vi "Datasheet Find Data.vi"(5 "SN":string, 6 "Test Type":string, 7 "MN":string, 8 "error in (no error)":errorcluster, 10 "Run Information":T2, 11 "Column Data":T1) -> (0 "error out":errorcluster, 3 "Column Item":string)   [LabVIEW 2011]
uses:
  TDMS/TDMS Run.ctl
  TDMS/TDMS Channel (Sxx).ctl
  database/Fields/Field Record.ctl
  database/Fields/Field DataTypes.ctl
  database/Fields/Field NextItem.ctl
  Column Data.ctl
  www/tests/S Parameter/TypeDefs/SP Format.ctl
  Datasheet Table Sxx Type.ctl
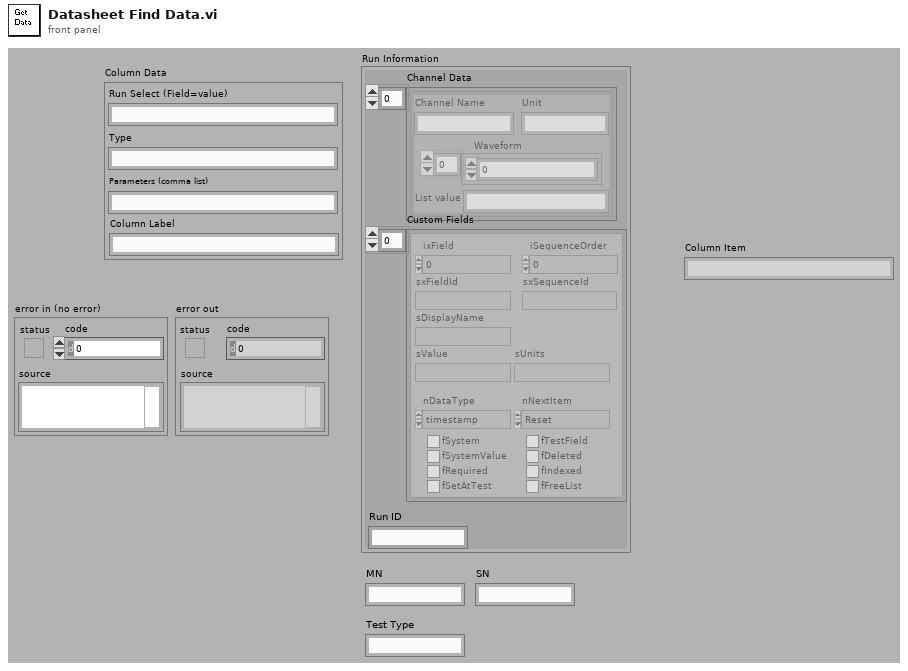
[diagram p1: front panel]
types:
  T1 = typedef "Column Data.ctl" = cluster{"Run Select (Field=value)":string, "Type":string, "Parameters (comma list)":string, "Column Label":string}
  T2 = typedef "TDMS Run.ctl" = cluster{"Channel Data":T3[], "Custom Fields":T4[], "Run ID":string}
  T3 = typedef "TDMS Channel (Sxx).ctl" = cluster{"Channel Name":string, "Waveform":dbl[], "Unit":string, "List value":string}
  T4 = typedef "Field Record.ctl" = cluster{"ixField":i32, "iSequenceOrder":i32, "sxFieldId":string, "sxSequenceId":string, "sDisplayName":string, "sValue":string, "sUnits":string, "nDataType":T5, "nNextItem":T6, "fSystem":bool, "fSystemValue":bool, "fRequired":bool, "fSetAtTest":bool, "fTestField":bool, "fDeleted":bool, "fIndexed":bool, "fFreeList":bool}
  T5 = typedef "Field DataTypes.ctl" = enum32{"text", "numeric", "list", "timestamp", "boolean"}
  T6 = typedef "Field NextItem.ctl" = enum32{"Reset", "Retain", "Auto-Increment"}
  T7 = typedef "datasheet table Sxx type.ctl" = enum16{"Value", "Maximum", "Minimum", "Max Freq", "maxlimit", "minlimit", "Min Freq", "maxfreqlimit", "minfreqlimit"}
  T8 = typedef "SP Format.ctl" = enum16{"Log Mag", "Lin Mag", "SWR", "Phase", "Expanded Phase", "Delay", "Insertion Loss", "Isolation", "Return Loss"}
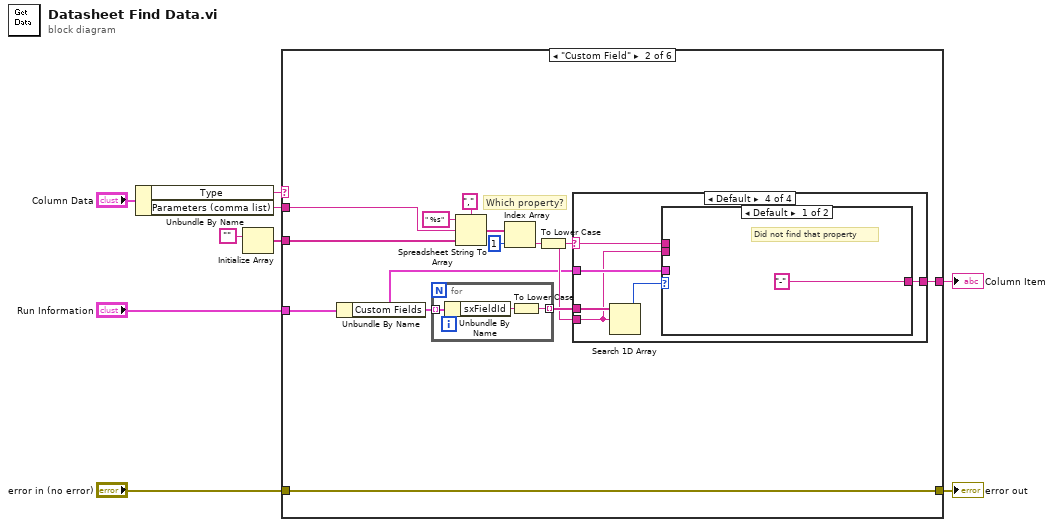
[diagram p0: block diagram]
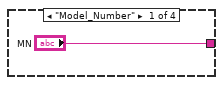
[diagram p3: hidden frame]
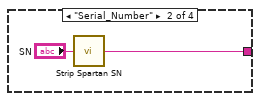
[diagram p4: hidden frame]
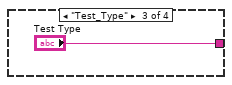
[diagram p5: hidden frame]
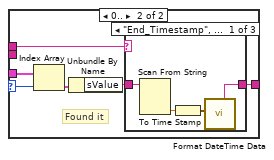
[diagram p6: hidden frame]
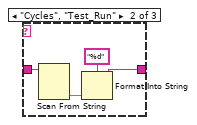
[diagram p7: hidden frame]
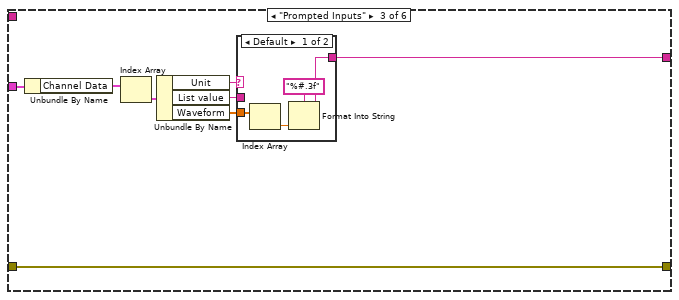
[diagram p9: hidden frame]
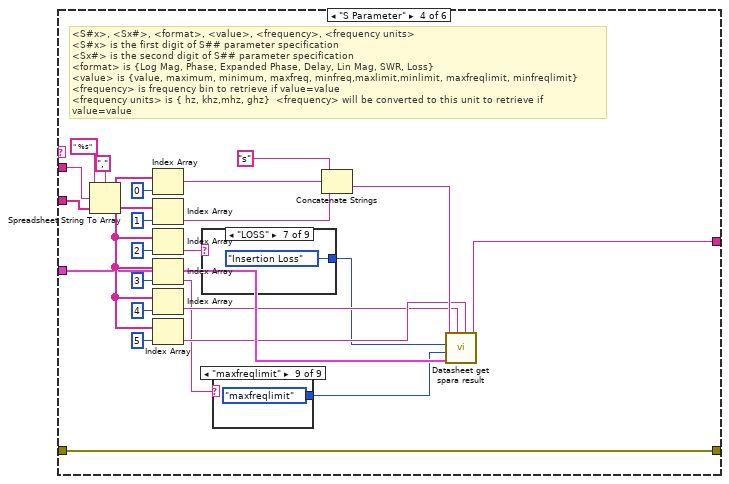
[diagram p11: hidden frame]
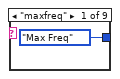
[diagram p12: hidden frame]
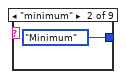
[diagram p13: hidden frame]
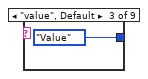
[diagram p14: hidden frame]
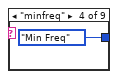
[diagram p15: hidden frame]
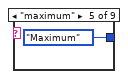
[diagram p16: hidden frame]
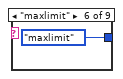
[diagram p17: hidden frame]
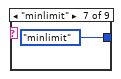
[diagram p18: hidden frame]
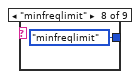
[diagram p19: hidden frame]
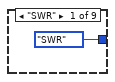
[diagram p20: hidden frame]
diagram:
  n1 = Unbundle By Name("Column Data") -> ("Type"=w8:string, "Parameters (comma list)"=w7:string)
  n2 = Initialize Array("") -> (w6:string[])  [unwired: 1 out]
  n3 = case shown="\"Custom Field\"" w8 {
    tunnel: w7 -> [w11 w21 _ w89 w121 w133]
    tunnel: w6 -> [_ w20 _ w88 w120 w132]
    tunnel: "Run Information" -> [_ w19 w60 w84 w109 w131]
    tunnel: [w11 w17 w55 w83 w116 w128] -> w3
    tunnel: "error in (no error)" -> [w10 w15 w61 w86 w118 w125]
    tunnel: [w10 w15 w61 w86 w118 w125] -> w1
    frame Default {
    }
    frame "Custom Field" {
      # "Which property?"
      n4 = Unbundle By Name(w19) -> ("Custom Fields"=w12:T4[])
      n5 = for {
        tunnel: w12 -> [w53] mode=indexing
        tunnel: [w51] -> w18 mode=indexing
        n6 = Unbundle By Name(w53) -> ("sxFieldId"=w52:string)
        n7 = To Lower Case(string=w52) -> (all lower case string=w51:string)
      }
      n8 = Spreadsheet String To Array(delimiter (Tab)=",", format string=" %s" ("delimiter (Tab)"), spreadsheet string=w21, array type (2D Dbl)=w20) -> (array=w22:string[])
      n9 = Index Array(array=w22, index=1) -> (element=w14:string)
      n10 = To Lower Case(string=w14) -> (all lower case string=w13:string)
      n11 = case shown="Default" w13 {
        selector: w13 -> [_ _ _ w29]
        tunnel: w18 -> [_ _ _ w34]
        tunnel: ["MN" w26 "Test Type" w32] -> w17
        tunnel: w12 -> [_ _ _ w31]
        tunnel: w13 -> [_ _ _ w30]
        frame "Model_Number" {
        }
        frame "Serial_Number" {
          n12 = call "Strip Spartan SN.vi"("SN 2"="SN") -> ("SN"=w26:string)
        }
        frame "Test_Type" {
        }
        frame Default {
          n13 = Search 1D Array(1D array=w34, element=w30) -> (index of element=w33:i32)  [unwired: 1 out]
          n14 = case shown="Default" w33 {
            selector: w33 -> [_ w40]
            tunnel: ["-" w36] -> w32
            tunnel: w31 -> [_ w41]
            tunnel: w30 -> [_ _]
            tunnel: w29 -> [_ w38]
            frame Default {
              # "Did not find that property"
            }
            frame 0.. {
              # "Found it"
              n15 = Index Array(array=w41, index=w40) -> (element=w39:T4)
              n16 = Unbundle By Name(w39) -> ("sValue"=w37:string)
              n17 = case shown="\"End_Timestamp\", \"Start_Timestamp\"" w38 {
                tunnel: [w42 w47 w50] -> w36
                tunnel: w37 -> [w45 w49 w50]
                frame "End_Timestamp", "Start_Timestamp" {
                  n18 = Scan From String(input string=w45) -> (output 1=w44:dbl)  [unwired: 3 in, 4 out]
                  n19 = To Time Stamp(1:w44) -> (0:w43:timestamp)
                  n20 = call "Format DateTime Data.vi"("Timestamp in"=w43) -> ("NON_UTC String out"=w42:string)  [unwired: 10 out]
                }
                frame "Cycles", "Test_Run" {
                  n21 = Scan From String(input string=w49) -> (output 1=w48:dbl)  [unwired: 3 in, 4 out]
                  n22 = Format Into String(format string="%d", w48) -> (resulting string=w47:string)  [unwired: 2 in, 1 out]
                }
                frame Default {
                }
              }
            }
          }
        }
      }
    }
    frame "Prompted Inputs" {
      n23 = Unbundle By Name(w60) -> ("Channel Data"=w59:T3[])
      n24 = Index Array(array=w59) -> (element=w58:T3)  [unwired: 1 in]
      n25 = Unbundle By Name(w58) -> ("Unit"=w57:string, "List value"=w56:string, "Waveform"=w54:dbl[])
      n26 = case shown="Default" w57 {
        tunnel: w56 -> [_ w66]
        tunnel: [w64 w66] -> w55
        tunnel: w54 -> [w63 _]
        frame Default {
          n27 = Index Array(array=w63) -> (element=w62:dbl)  [unwired: 1 in]
          n28 = Format Into String(format string="%#.3f", w62) -> (resulting string=w64:string)  [unwired: 2 in, 1 out]
        }
        frame "Enumeration" {
        }
      }
    }
    frame "S Parameter" {
      # "<S#x>, <Sx#>, <format>, <value>, <frequency>, <frequency units>\n<S#x> is the first digit of S## parameter specification\n<Sx#> is the second digit of S## parameter specification\n<format> is {Log Mag, Phase, Expanded Phase, Delay, Lin Mag, SWR, Loss}\n<value> is {value, maximum, minimum, maxfreq, minfreq,maxlimit,minlimit, maxfreqlimit, minfreqlimit}  \n<frequency> is frequency bin to retrieve if value=value\n<frequency units> is { hz, khz,mhz, ghz}  <frequency> will be converted to this unit to retrieve if value=value"
      n29 = Spreadsheet String To Array(delimiter (Tab)=",", format string=" %s" ("delimiter (Tab)"), spreadsheet string=w89, array type (2D Dbl)=w88) -> (array=w85:string[])
      n30 = Index Array(array=w85, index=0) -> (element=w75:string)
      n31 = Index Array(array=w85, index=1) -> (element=w76:string)
      n32 = Index Array(array=w85, index=2) -> (element=w68:string)
      n33 = Index Array(array=w85, index=3) -> (element=w67:string)
      n34 = Index Array(array=w85, index=4) -> (element=w71:string)
      n35 = Index Array(array=w85, index=5) -> (element=w72:string)
      n36 = case shown="\"LOSS\"" w68 {
        tunnel: [SP_Format."SWR" ("Format") SP_Format."Log Mag" ("Format") SP_Format."Lin Mag" ("Format") SP_Format."Phase" ("Format") SP_Format."Expanded Phase" ("Format") SP_Format."Delay" ("Format") SP_Format."Insertion Loss" ("Format") SP_Format."Isolation" ("Format") SP_Format."Return Loss" ("Format")] -> w69
        frame "SWR" {
        }
        frame "LOG MAG", Default {
        }
        frame "LIN MAG" {
        }
        frame "PHASE" {
        }
        frame "EXPANDED PHASE" {
        }
        frame "DELAY" {
        }
        frame "LOSS" {
        }
        frame "ISOLATION" {
        }
        frame "RETURN LOSS" {
        }
      }
      n37 = case shown="\"maxfreqlimit\"" w67 {
        tunnel: [datasheet_table_Sxx_type."Max Freq" ("Type") datasheet_table_Sxx_type."Minimum" ("Type") datasheet_table_Sxx_type."Value" ("Type") datasheet_table_Sxx_type."Min Freq" ("Type") datasheet_table_Sxx_type."Maximum" ("Type") datasheet_table_Sxx_type."maxlimit" ("Type") datasheet_table_Sxx_type."minlimit" ("Type") datasheet_table_Sxx_type."minfreqlimit" ("Type") datasheet_table_Sxx_type."maxfreqlimit" ("Type")] -> w70
        frame "maxfreq" {
        }
        frame "minimum" {
        }
        frame "value", Default {
        }
        frame "minfreq" {
        }
        frame "maximum" {
        }
        frame "maxlimit" {
        }
        frame "minlimit" {
        }
        frame "minfreqlimit" {
        }
        frame "maxfreqlimit" {
        }
      }
      n38 = Concatenate Strings("s" ("delimiter (Tab)"), w75, w76) -> (w73:string)
      n39 = call "Datasheet get spara result.vi"("Frequency unit"=w72, "Frequency"=w71, "Run Information"=w84, "Type"=w70, "Format"=w69, "Sxx"=w73) -> ("Table item"=w83:string)  [unwired: 5 out]
    }
    frame "PIM" {
      # "Parameter>,  <Units>, <Direction>\n\n<Parameter> = {MaximumIM, Carrier1, Carrier2, MaximumFreq, Mean, StandardDev, Transmit1, Transmit2, Samples, Limit}\n<Units> = {dBm, dBc, Hz, kHz, MHz, GHz}\n<Direction> = {Up, Down}"
      n40 = Spreadsheet String To Array(delimiter (Tab)=",", format string=" %s" ("delimiter (Tab)"), spreadsheet string=w121, array type (2D Dbl)=w120) -> (array=w117:string[])
      n41 = Index Array(array=w117, index=0) -> (element=w112:string)
      n42 = Index Array(array=w117, index=1) -> (element=w111:string)
      n43 = Index Array(array=w117, index=2) -> (element=w110:string)
      n44 = call "Datasheet get PIM result.vi"("Run Information"=w109, "DIRECTION"=w110, "UNITS"=w111, "PARAMETER"=w112) -> ("Table item"=w116:string)  [unwired: 1 in, 6 out]
    }
    frame "DC Attenuation" {
      # "R2"
      # "Which channel"
      n45 = Unbundle By Name(w131) -> ("Channel Data"=w127:T3[])
      n46 = Spreadsheet String To Array(delimiter (Tab)=",", format string=" %s" ("delimiter (Tab)"), spreadsheet string=w133, array type (2D Dbl)=w132) -> (array=w134:string[])
      n47 = Index Array(array=w134, index=0) -> (element=w123:string)
      n48 = for {
        tunnel: w127 -> [w149] mode=indexing
        tunnel: [w147] -> w130 mode=indexing
        n49 = Unbundle By Name(w149) -> ("Channel Name"=w148:string)
        n50 = To Lower Case(string=w148) -> (all lower case string=w147:string)
      }
      n51 = To Lower Case(string=w123) -> (all lower case string=w124:string)
      n52 = Search 1D Array(1D array=w130, element=w124) -> (index of element=w129:i32)  [unwired: 1 out]
      n53 = case shown="0.." w129 {
        selector: w129 -> [_ w145]
        tunnel: [w138 w141] -> w128
        tunnel: w127 -> [_ w146]
        tunnel: w124 -> [w137 _]
        frame Default {
          # "Did not find that property"
          n54 = Concatenate Strings("Missing Channel -", w137) -> (w138:string)
        }
        frame 0.. {
          # "Found it"
          n55 = Index Array(array=w146, index=w145) -> (element=w144:T3)
          n56 = Unbundle By Name(w144) -> ("Waveform"=w143:dbl[])
          n57 = Index Array(array=w143) -> (element=w142:dbl)  [unwired: 1 in]
          n58 = Format Into String(format string="%#.3f", w142) -> (resulting string=w141:string)  [unwired: 2 in, 1 out]
        }
      }
    }
  }
  "Column Item" <- w3
  "error out" <- w1
